vi "VOLTAGE.vi"(7 "error in (no error)":errorcluster, 9 "Voltage Limit":dbl=1.0, 10 "VISA resource name":refnum<visa-resource-name>) -> (0 "error out":errorcluster, 1 "Read out result":string="UC= 9456.092   PF L= 658.76     NS V=0.10   V\r\n", 2 "Send string":string="UNITS 1;\nSHOW UN", 3 "VISA resource name out":refnum<visa-resource-name>)   [LabVIEW 2019, in "AH2500.lvlib"]
uses:
  AH2500.lvlib
panel:
  # "Set the highest AC voltage limit"
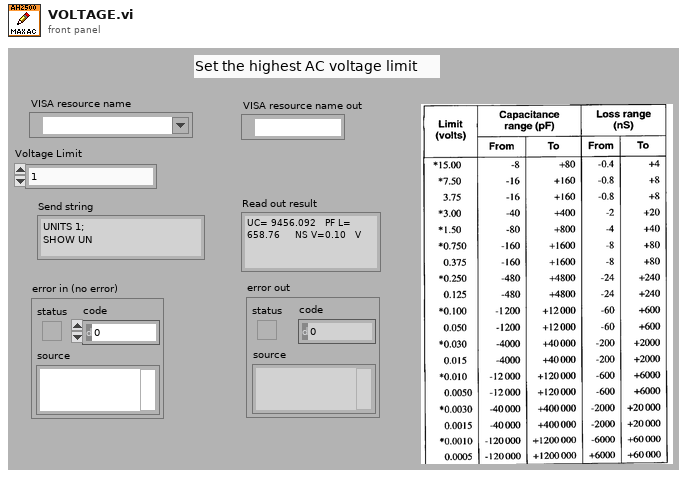
[diagram p1: front panel]
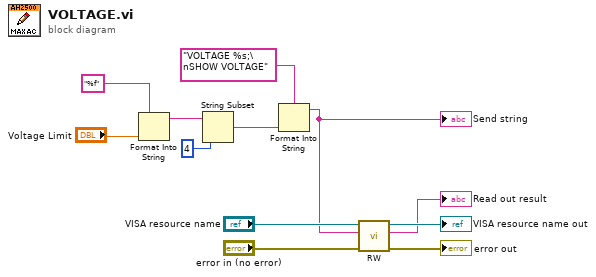
[diagram p0: block diagram]
diagram:
  n1 = Format Into String(format string="%f", "Voltage Limit") -> (resulting string=w10:string)  [unwired: 2 in, 1 out]
  n2 = String Subset(string=w10, length (rest)=4 ("length (rest)")) -> (substring=w7:string)  [unwired: 1 in]
  n3 = Format Into String(format string="VOLTAGE %s;\nSHOW VOLTAGE", w7) -> (resulting string=w5:string)  [unwired: 2 in, 1 out]
  "Send string" <- w5
  n4 = call "RW.vi"("error in (no error)"="error in (no error)", "write buffer"=w5, "VISA Refnum in"="VISA resource name") -> ("error out"=→"error out":errorcluster, "read buffer"=→"Read out result":string, "VISA Refnum out"=→"VISA resource name out":refnum<visa-resource-name>)  [unwired: 6 in]
